vi "RSZVB Set Time Domain Time Axis Scaling.vi"(8 "error in (no error)":errorcluster {"code" format="%.0x"}, 9 "Time Axis Scaling (1: Time)":i32(ring)=1 items=["Distance", "Time"], 10 "Channel (Trace) (1)":i32=1, 11 "VISA session":refnum<visa-resource-name>) -> (0 "error out":errorcluster {"code" format="%.0x"}, 3 "dup VISA session":refnum<visa-resource-name>)   [LabVIEW 2011]
doc: "This VI switches over between the x-axis scaling in time units or distance units.\n\nRemote-control command(s):\nCALCulate<Ch/Tr>:TRANsform:TIME:XAXis TIME | DISTance"
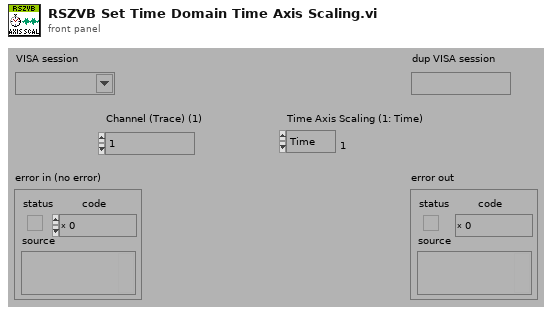
[diagram p1: front panel]
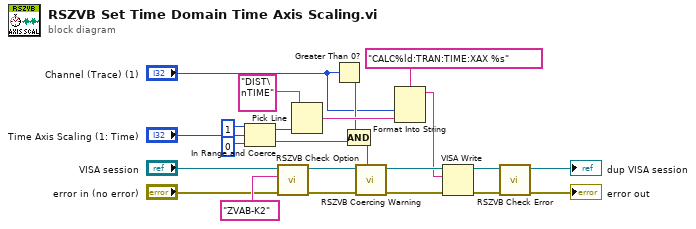
[diagram p0: block diagram]
diagram:
  n1 = In Range and Coerce(upper limit=1, x="Time Axis Scaling (1: Time)", lower limit=0) -> (coerced(x)=w10:i32, In Range?=w13:bool)
  n2 = call "RSZVB Check Option.vi"("error in (no error)"="error in (no error)", "Options"="ZVAB-K2", "VISA session"="VISA session") -> ("error out"=w9:errorcluster, "dup VISA session"=w8:refnum<visa-resource-name>)  [unwired: 7 in]
  n3 = Pick Line(multi-line string="DIST\nTIME", line index=w10) -> (output string=w16:string)  [unwired: 1 in]
  n4 = Greater Than 0?(x="Channel (Trace) (1)") -> (x > 0?=w12:bool)
  n5 = Compound Arithmetic op=AND(w12, w13) -> (w11:bool)
  n6 = call "RSZVB Coercing Warning.vi"("In Range?"=w11, "error in (no error)"=w9, "VISA session"=w8) -> ("error out"=w21:errorcluster, "dup VISA session"=w22:refnum<visa-resource-name>)  [unwired: 7 in]
  n7 = Format Into String(format string="CALC%ld:TRAN:TIME:XAX %s", "Channel (Trace) (1)", w16) -> (resulting string=w18:string)  [unwired: 2 in, 1 out]
  n8 = VISA Write(VISA resource name=w22, write buffer=w18, error in (no error)=w21) -> (VISA resource name out=w19:refnum<visa-resource-name>, error out=w20:errorcluster)  [unwired: 1 out]
  n9 = call "RSZVB Check Error.vi"("error in (no error)"=w20, "VISA session"=w19) -> ("error out"=→"error out":errorcluster, "dup VISA session"=→"dup VISA session":refnum<visa-resource-name>)  [unwired: 8 in]
